vi "Periodic Tasks.vi"(8 "error in":errorcluster) -> ()   [LabVIEW 2019]
doc: "This VI runs in parallel to other tasks. It can contain as many user-defined periodic loops as you need. These can carry out PID or other sorts of timed response."
uses:
  <vilib>/Rock Robotics/WPI/DriverStation/WPI_DriverStationRobotMode2.ctl
  <vilib>/Rock Robotics/WPI/Utilities/WPI_GetSetVariantRefNum.vi
  Robot Global Data.vi
  <vilib>/Rock Robotics/Network Tables/NT Write Number.vi
  <vilib>/Rock Robotics/Network Tables/NT Write Boolean.vi
  <vilib>/Rock Robotics/WPI/RobotDrive/WPI_RobotDriveArcadeDrive_Standard(NoSaturation).vi
  <vilib>/Rock Robotics/Network Tables/NT Write Numeric Array.vi
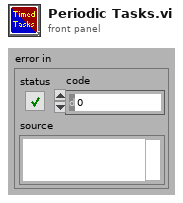
[diagram p1: front panel]
types:
  T1 = typedef "WPI_JoystickDevRef.ctl" = cluster{"Device":T2}
  T2 = typedef "WPI_JoystickDeviceEnum.ctl" = enum16{"USB 0", "USB 1", "USB 2", "USB 3", "USB 4", "USB 5"}
  T3 = typedef "WPI_RobotDriveDevRef.ctl" = cluster{"DevStatus":errorcluster, "Motors[]":T4[], "Square Inputs":bool, "Max Output":dbl}
  T4 = typedef "WPI_MotorControlDeviceRef.ctl" = cluster{"DeviceStatus":errorcluster, "Type":T5, "PWM":cluster{"PWM Channel":T6, "DeadBand":T7}, "CAN":cluster{"Device Number":u8, "SetOutput VI Ref":variant, "GetOutput VI Ref":variant, "Enable VI Ref":variant, "Disable VI Ref":variant, "Data":variant}, "Invert":bool, "DIO PWM":cluster{"PWM \"Enable\" Channel":T6, "DIOChannel":T8, "PWM Rate":dbl}}
  T5 = typedef "WPI_MotorControlType.ctl" = enum16{"PWM", "CAN", "DIO PWM"}
  T6 = typedef "FPGA_DIOPWMChannel.ctl" = enum8{"PWM 0", "PWM 1", "PWM 2", "PWM 3", "PWM 4", "PWM 5", "PWM 6", "PWM 7", "PWM 8", "PWM 9", "PWM MXP 0", "PWM MXP 1", "PWM MXP 2", "PWM MXP 3", "PWM MXP 4", "PWM MXP 5", "PWM MXP 6", "PWM MXP 7", "PWM MXP 8", "PWM MXP 9", "Invalid"}
  T7 = typedef "WPI_PWMDeadband.ctl" = cluster{"Name":string, "maxPositivePwm":i32, "minPositivePwm":i32, "centerPwm":i32, "maxNegativePwm":i32, "minNegativePwm":i32, "angularRange":u16}
  T8 = typedef "FPGA_DIOChannel.ctl" = enum8{"DIO 0", "DIO 1", "DIO 2", "DIO 3", "DIO 4", "DIO 5", "DIO 6", "DIO 7", "DIO 8", "DIO 9", "DIO MXP 0", "DIO MXP 1", "DIO MXP 2", "DIO MXP 3", "DIO MXP 4", "DIO MXP 5", "DIO MXP 6", "DIO MXP 7", "DIO MXP 8", "DIO MXP 9", "DIO MXP 10", "DIO MXP 11", "DIO MXP 12", "DIO MXP 13", "DIO MXP 14", "DIO MXP 15", "SPI Port CS1", "SPI Port CS2", "SPI Port CS3", "SPI Port MISO", "SPI Port MOSI", "Invalid"}
  T9 = cluster{"JoystickDevRef":T1, "RobotDriveDevRef":T3}
  T10 = typedef "WPI_DriverStationRobotMode2.ctl" = enum16{"Autonomous Disabled", "Autonomous Enabled", "Teleop Disabled", "Teleop Enabled", "Disconnected", "Finish", "Test Disabled", "Test Enabled", "Emergency Stopped"}
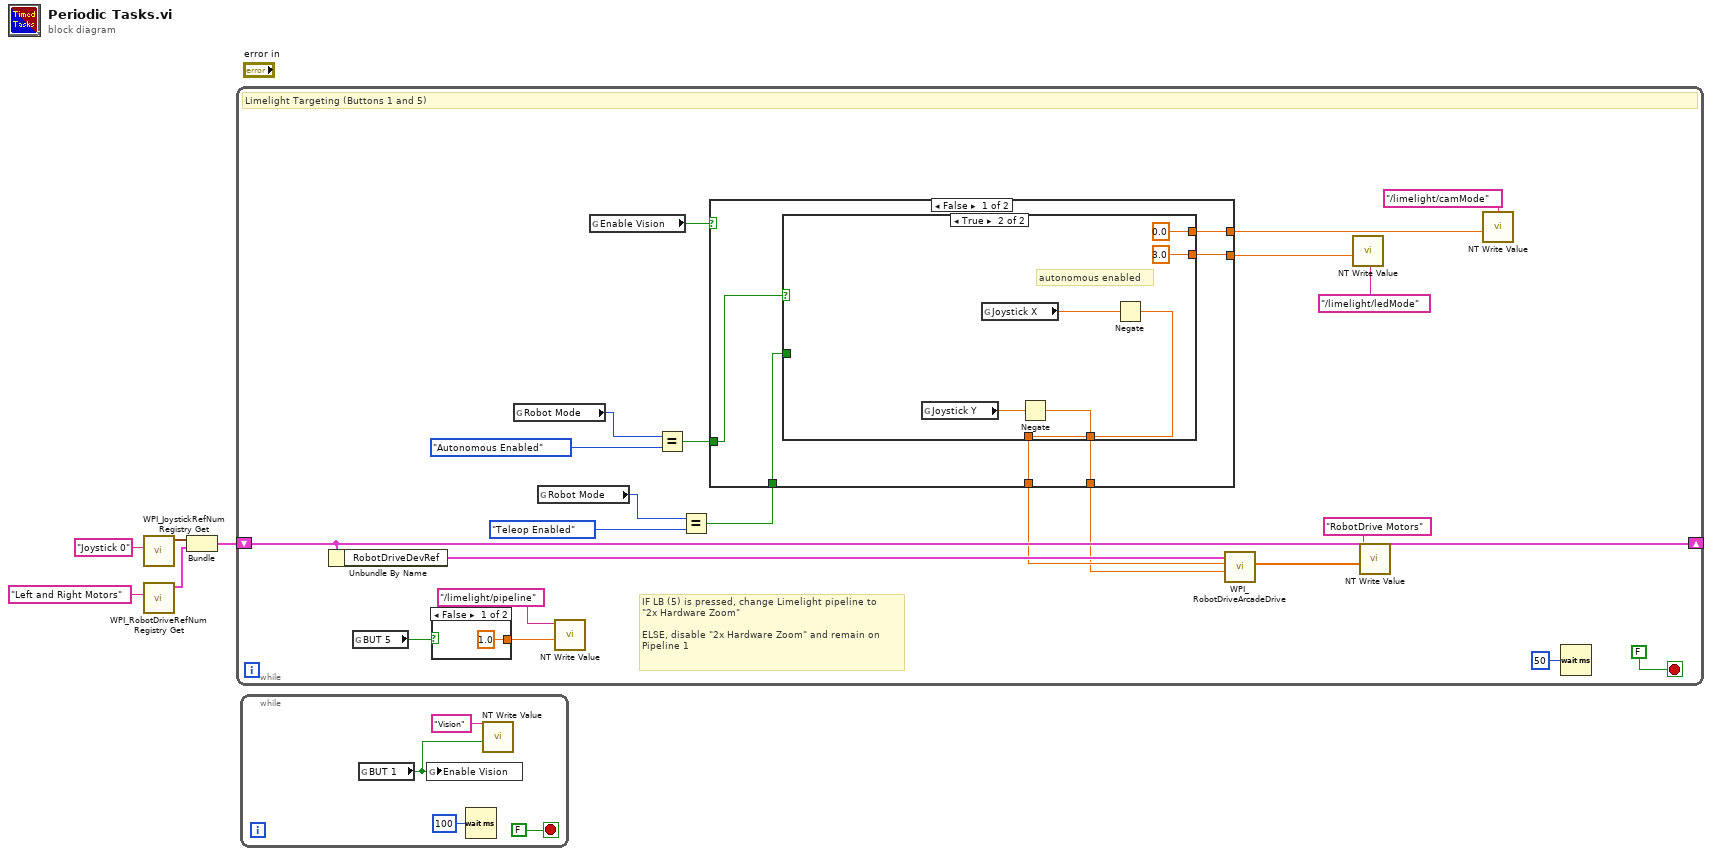
[diagram p0: block diagram]
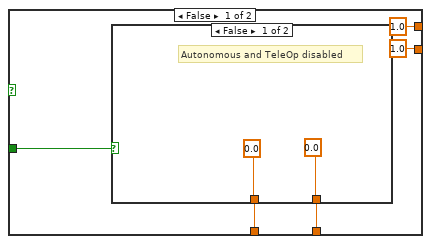
[diagram p2: hidden frame]
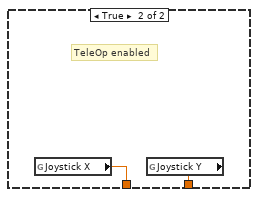
[diagram p3: hidden frame]
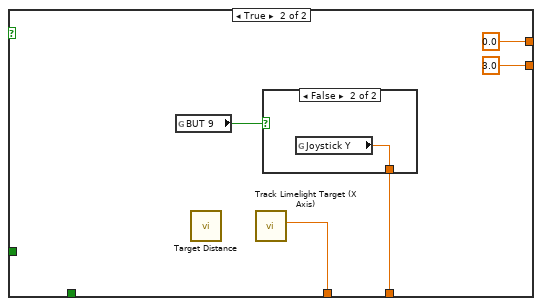
[diagram p4: hidden frame]
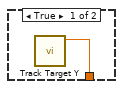
[diagram p5: hidden frame]
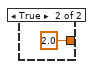
[diagram p6: hidden frame]
diagram:
  n1 = call <vilib>:"WPI_JoystickRefNum Registry Get.vi"("refnum name"="Joystick 0") -> ("JoystickDevRef"=w3:T1)  [unwired: 1 in, 9 out]
  n2 = call <vilib>:"WPI_RobotDriveRefNum Registry Get.vi"("refnum name"="Left and Right Motors") -> ("RobotDriveDevRef"=w2:T3)  [unwired: 1 in, 9 out]
  n3 = Bundle("JoystickDevRef"=w3, "RobotDriveDevRef"=w2) -> (w1:T9)  [unwired: 1 out]
  n4 = while {
    shift-right: [w26] -> _
    shift-left: w1 -> [w26]
    stop <- FALSE stop-if-true
    # "IF LB (5) is pressed, change Limelight pipeline to \n\"2x Hardware Zoom\"\n\nELSE, disable \"2x Hardware Zoom\" and remain on\nPipeline 1"
    # "Limelight Targeting (Buttons 1 and 5)"
    n5 = Unbundle By Name(w26) -> ("RobotDriveDevRef"=w23:T3)
    n6 = global read "Robot Global Data.vi" "BUT 5"() -> (w8:bool)
    n7 = case shown="False" w8 {
      tunnel: [1.0 ("Numeric") 2.0 ("Numeric")] -> w22
      frame False {
      }
      frame True {
      }
    }
    n8 = global read "Robot Global Data.vi" "Robot Mode"() -> (w17:T10)
    n9 = global read "Robot Global Data.vi" "Robot Mode"() -> (w13:T10)
    n10 = call-poly <vilib>:"NT Write Value.vi"("Numeric"=w22, "Name"="/limelight/pipeline") -> ()  [unwired: 9 in, 1 out]
    n11 = global read "Robot Global Data.vi" "Enable Vision"() -> (w9:bool)
    n12 = Equal?(x=w17, y=WPI_DriverStationRobotMode2."Autonomous Enabled") -> (x = y?=w15:bool)
    n13 = Equal?(x=w13, y=WPI_DriverStationRobotMode2."Teleop Enabled") -> (x = y?=w12:bool)
    n14 = case shown="False" w9 {
      tunnel: [w30 0.0 ("Numeric")] -> w19
      tunnel: [w29 3.0 ("Numeric")] -> w18
      tunnel: [w33 w51] -> w10
      tunnel: w15 -> [w31 _]
      tunnel: w12 -> [w32 _]
      tunnel: [w28 w50] -> w11
      frame False {
        n15 = case shown="True" w31 {
          tunnel: [w37 w47] -> w33
          tunnel: [w38 w46] -> w28
          tunnel: w32 -> [w36 _]
          tunnel: [1.0 ("Numeric") 0.0 ("Numeric")] -> w30
          tunnel: [1.0 ("Numeric") 3.0 ("Numeric")] -> w29
          frame False {
            n16 = case shown="False" w36 {
              tunnel: [0.0 ("Joystick X") w42] -> w38
              tunnel: [0.0 ("Joystick Y") w41] -> w37
              frame False {
                # "Autonomous and TeleOp disabled"
              }
              frame True {
                # "TeleOp enabled"
                n17 = global read "Robot Global Data.vi" "Joystick X"() -> (w42:dbl)
                n18 = global read "Robot Global Data.vi" "Joystick Y"() -> (w41:dbl)
              }
            }
          }
          frame True {
            # "autonomous enabled"
            n19 = global read "Robot Global Data.vi" "Joystick Y"() -> (w48:dbl)
            n20 = global read "Robot Global Data.vi" "Joystick X"() -> (w45:dbl)
            n21 = Negate(x=w48) -> (-x=w47:dbl)
            n22 = Negate(x=w45) -> (-x=w46:dbl)
          }
        }
      }
      frame True {
        n23 = global read "Robot Global Data.vi" "BUT 9"() -> (w49:bool)
        n24 = call "Target Distance.vi"() -> ()  [unwired: 12 in]
        n25 = call "Track Limelight Target (X Axis).vi"() -> ("Joystick X"=w50:dbl)  [unwired: 11 in]
        n26 = case shown="False" w49 {
          tunnel: [w54 w55] -> w51
          frame True {
            n27 = call "Track Target Y.vi"() -> ("Joystick Y"=w54:dbl)  [unwired: 11 in]
          }
          frame False {
            n28 = global read "Robot Global Data.vi" "Joystick Y"() -> (w55:dbl)
          }
        }
      }
    }
    n29 = call-poly <vilib>:"WPI_RobotDriveArcadeDrive.vi"("Y axis value"=w10, "X axis value"=w11, "RobotDriveDevRef"=w23) -> ("Motor Values"=w6:dbl[])  [unwired: 6 in, 2 out]
    n30 = call-poly <vilib>:"NT Write Value.vi"("Numeric"=w18, "Name"="/limelight/ledMode" ("LED Mode")) -> ()  [unwired: 9 in, 1 out]
    n31 = call-poly <vilib>:"NT Write Value.vi"("Numeric Array"=w6, "Name"="RobotDrive Motors") -> ()  [unwired: 9 in, 1 out]
    n32 = call-poly <vilib>:"NT Write Value.vi"("Numeric"=w19, "Name"="/limelight/camMode" ("Camera Mode")) -> ()  [unwired: 9 in, 1 out]
    n33 = Wait (ms)(milliseconds to wait=u32 50) -> ()  [unwired: 1 out]
  }
  n34 = while {
    stop <- FALSE stop-if-true
    n35 = global read "Robot Global Data.vi" "BUT 1"() -> (w58:bool)
    n36 = global write "Robot Global Data.vi" "Enable Vision"(w58) -> ()
    n37 = Wait (ms)(milliseconds to wait=u32 100) -> ()  [unwired: 1 out]
    n38 = call-poly <vilib>:"NT Write Value.vi"("Boolean"=w58, "Name"="Vision") -> ()  [unwired: 9 in, 1 out]
  }
